vi "test - csm RCM dependencies.vi"(8 "error in (no error)":errorcluster, 11 "TestCase in":refnum<class "testcase-documentation.lvclass">) -> (0 "error out":errorcluster, 3 "TestCase out":refnum<class "testcase-documentation.lvclass">)   [LabVIEW 2017, in "testcase-documentation.lvclass"]
uses:
  testcase-documentation.lvclass
  <vilib>/addons/_JKI Toolkits/VI Tester/TestCase.llb/TestCase.lvclass
  src/user.lib/_NEVSTOP/Communicable State Machine(CSM)/Communicable State Machine.lvlib
  C:/Program Files (x86)/National Instruments/LabVIEW 2017/vi.lib/addons/_JKI Toolkits/VI Tester/TestCase.llb/TestCase.lvclass
panel:
  out "Dependency Paths 2":path[](array[path])
  out "Dependency Paths":string[](array[string])
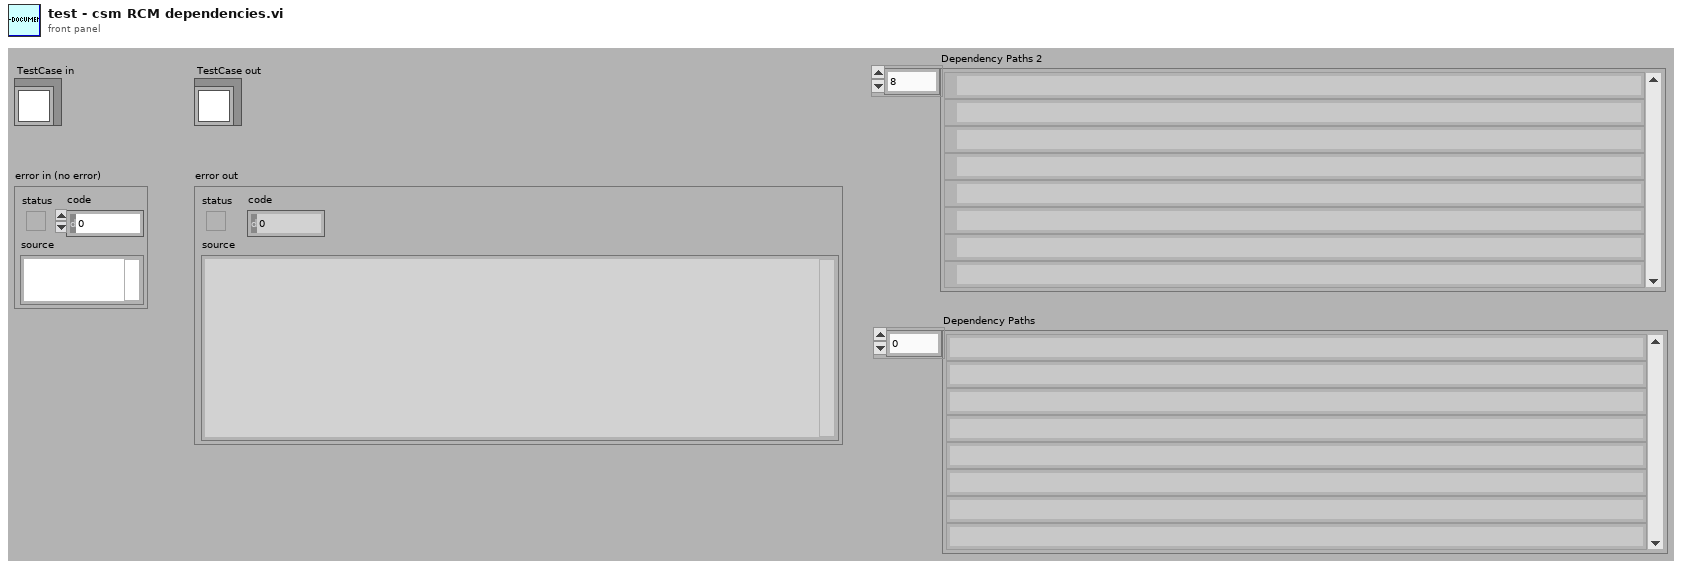
[diagram p1: front panel]
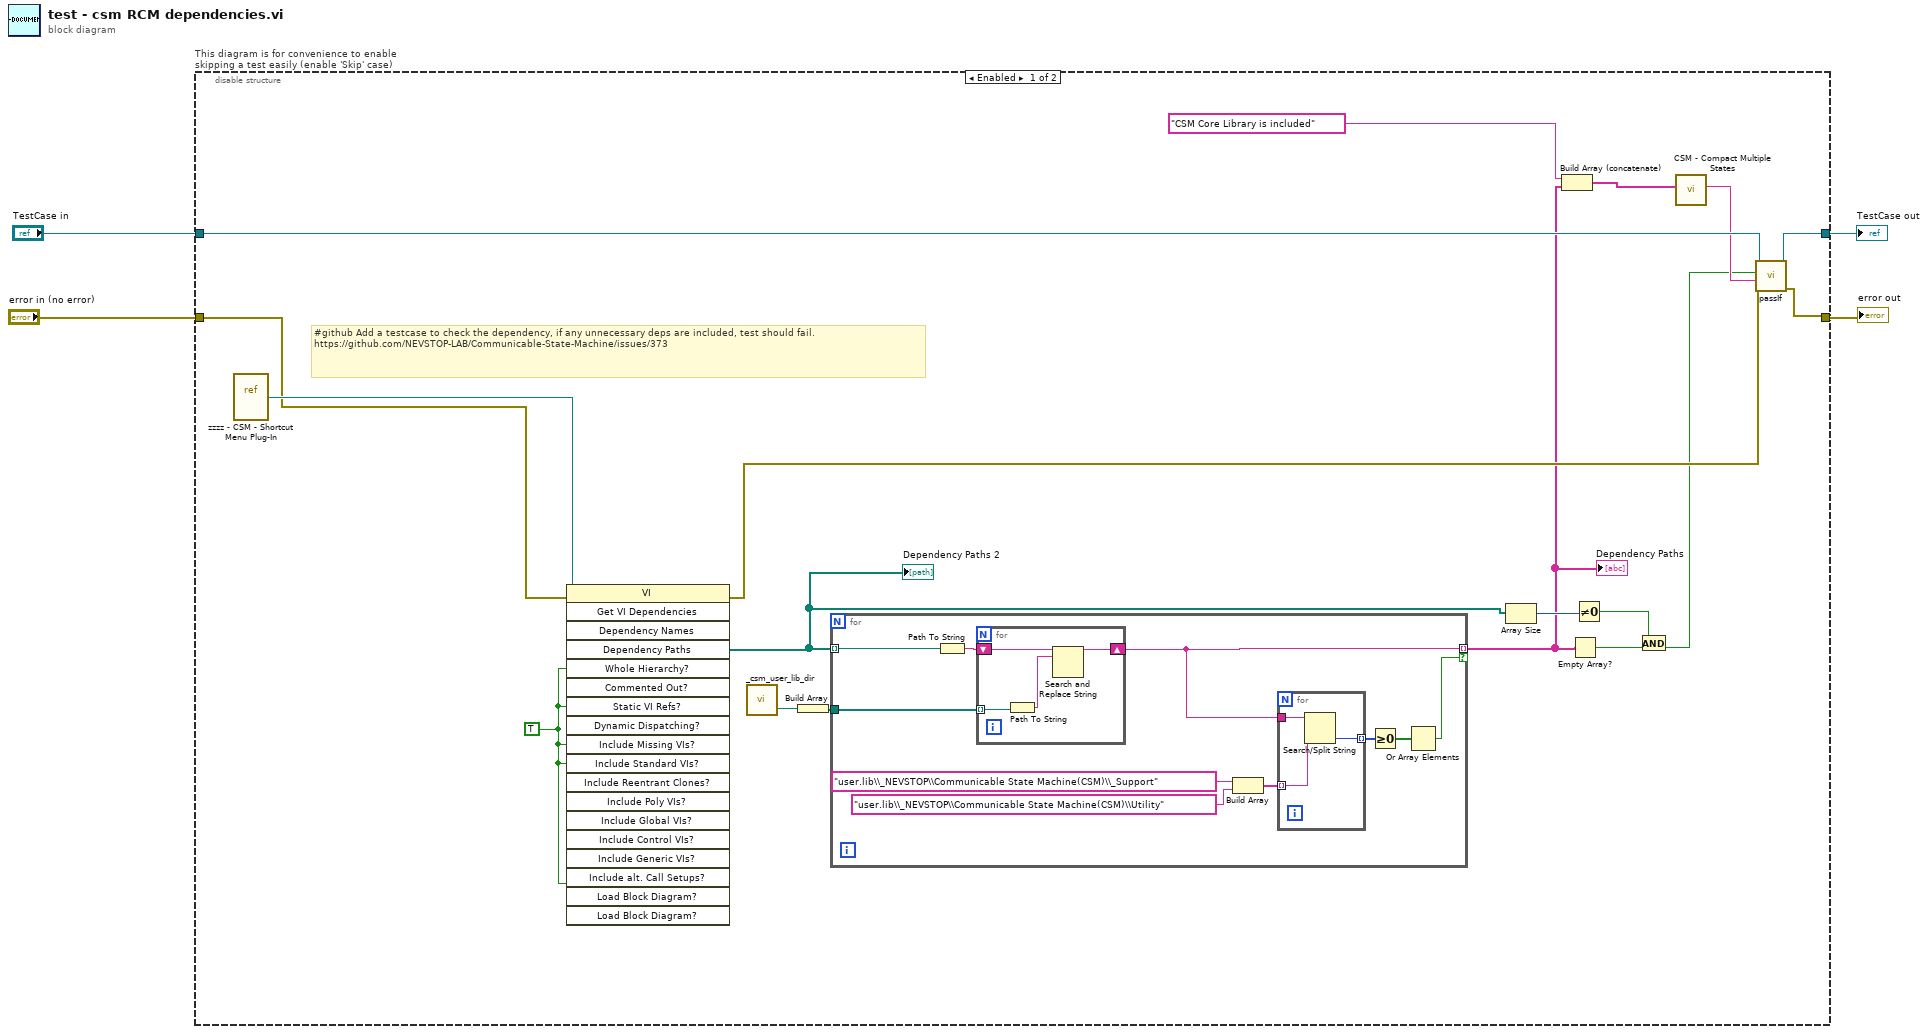
[diagram p0: block diagram]
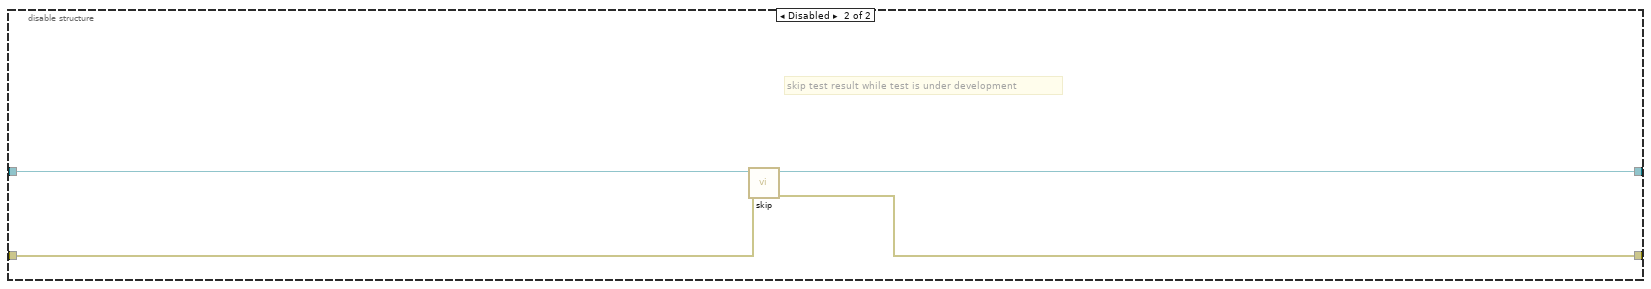
[diagram p2: hidden frame]
diagram:
  n1 = disable-structure "This diagram is for convenience to enable skipping a test easily (enable 'Skip' case)" shown="Enabled" {
    disable-tunnel: "TestCase in" -> [w22 w43]
    disable-tunnel: [w21 w41] -> w1
    disable-tunnel: [w20 w42] -> w3
    disable-tunnel: "error in (no error)" -> [w7 w40]
    frame Enabled {
      w16 = TRUE ("Include Missing Items?")
      # "#github Add a testcase to check the dependency, if any unnecessary deps are included, test should fail. \nhttps://github.com/NEVSTOP-LAB/Communicable-State-Machine/issues/373"
      n2 = vi-ref "zzzz - CSM - Shortcut Menu Plug-In.vi"() -> (w8:refnum<vi>)
      n3 = invoke class="VI" method="Get VI Dependencies"(reference=w8, error in=w7, "Whole Hierarchy?"=w16, "Static VI Refs?"=w16, "Include Missing VIs?"=w16, "Include Standard VIs?"=w16, "Include Poly VIs?"=w16, "Include Global VIs?"=w16, "Include Control VIs?"=w16, "Include Generic VIs?"=w16, "Include alt. Call Setups?"=w16) -> (error out=w15:errorcluster, "Dependency Paths"=w5:path[])  [unwired: 8 in, 17 out]
      "Dependency Paths 2" <- w5
      n4 = call "_csm_user_lib_dir.vi"() -> ("<LabVIEW>"=w9:path)  [unwired: 2 in, 1 out]
      n5 = Build Array(w9) -> (w10:path[])
      n6 = for {
        tunnel: w5 -> [w32] mode=indexing
        tunnel: w10 -> [w30]
        tunnel: [w23] -> w6 mode=indexing if=w24
        n7 = Path To String(path=w32) -> (string=w31:string)
        n8 = for {
          tunnel: w30 -> [w38] mode=indexing
          shift-right: [w36] -> w23
          shift-left: w31 -> [w39]
          n9 = Path To String(path=w38) -> (string=w37:string)
          n10 = Search and Replace String(input string=w39, search string=w37) -> (result string=w36:string)  [unwired: 6 in, 3 out]
        }
        n11 = Build Array("user.lib\\_NEVSTOP\\Communicable State Machine(CSM)\\_Support" ("regular expression"), "user.lib\\_NEVSTOP\\Communicable State Machine(CSM)\\Utility" ("regular expression")) -> (w26:string[])
        n12 = for {
          tunnel: w23 -> [w35]
          tunnel: [w34] -> w28 mode=indexing
          tunnel: w26 -> [w33] mode=indexing
          n13 = Search/Split String(string=w35, search string/char (-)=w33) -> (offset of match=w34:i32)  [unwired: 1 in, 2 out]
        }
        n14 = Greater Or Equal To 0?(x=w28) -> (x >= 0?=w27:bool[])
        n15 = Or Array Elements(Boolean array=w27) -> (logical OR=w24:bool)
      }
      "Dependency Paths" <- w6
      n16 = Array Size(array=w5) -> (size(s)=w12:i32)
      n17 = Build Array (concatenate)("CSM Core Library is included" ("message (\"\")"), w6) -> (w19:string[])
      n18 = Empty Array?(array=w6) -> (empty?=w11:bool)
      n19 = Not Equal To 0?(x=w12) -> (x != 0?=w13:bool)
      n20 = And(x=w13, y=w11) -> (x .and. y?=w14:bool)
      n21 = call "CSM - Compact Multiple States.vi"("Multiple States"=w19) -> ("States"=w18:string)  [unwired: 9 in]
      n22 = call-dynamic "passIf.vi"("error in (no error)"=w15, "message (\"\")"=w18, "pass"=w14, "TestCase in"=w22) -> ("error out"=w20:errorcluster, "TestCase out"=w21:refnum<class "testcase-documentation.lvclass">)  [unwired: 6 in]
    }
    frame Disabled {
      # "skip test result while test is under development"
      n23 = call <vilib>:"skip.vi"("error in (no error)"=w40, "TestCase in"=w43) -> ("error out"=w42:errorcluster, "TestCase out"=w41:refnum<class "testcase-documentation.lvclass">)  [unwired: 8 in]
    }
  }
  "error out" <- w3
  "TestCase out" <- w1
